vi "ToModelQueue_bac.vi"(7 "Enum":T1, 8 "error in (no error)":errorcluster) -> (0 "error out":errorcluster, 3 "queue out":refnum<queue>)   [LabVIEW 2021]
uses:
  QueueEnum.ctl
  ModelQueueCluster.ctl
  ToModelSourceEnum.ctl
  FromTCPCluster.ctl
  ToModelFromTCPMessage.ctl
  FormControllerToMOdelCluster.ctl
  ToModelFromControllerEnum.ctl
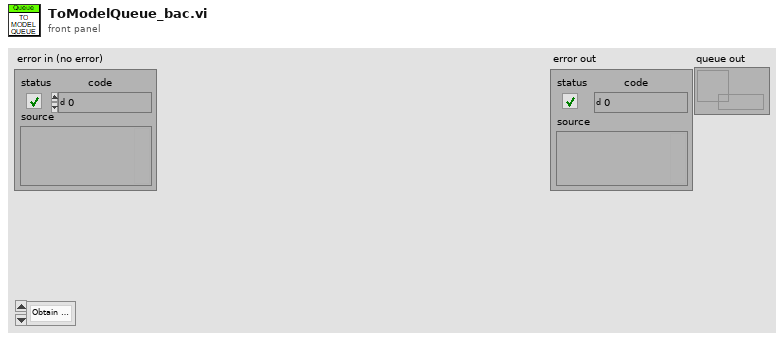
[diagram p1: front panel]
types:
  T1 = typedef "QueueEnum.ctl" = enum16{"Obtain Queue", "Get Queue Ref", "Flush Queue", "Release Queue"}
  T2 = typedef "ModelQueueCluster.ctl" = cluster{T3, "FromTCPCluster":T4, "FromControllerCluster":T6}
  T3 = typedef "ToModelSourceEnum.ctl" = enum16{"TCP", "Controller"}
  T4 = typedef "FromTCPCluster.ctl" = cluster{"Message":T5, "Data":string, "StatusOK?":bool}
  T5 = typedef "ToModelFromTCPMessage.ctl" = enum16{"Exit", "DataWritten", "DataReceived", "Timeout", "UnableToConnect", "Disconnected", "Connected"}
  T6 = typedef "FormControllerToMOdelCluster.ctl" = cluster{"Enum":T7, "IP Address":string, "Remote Port":u16}
  T7 = typedef "ToModelFromControllerEnum.ctl" = enum16{"Disconnect", "Connect"}
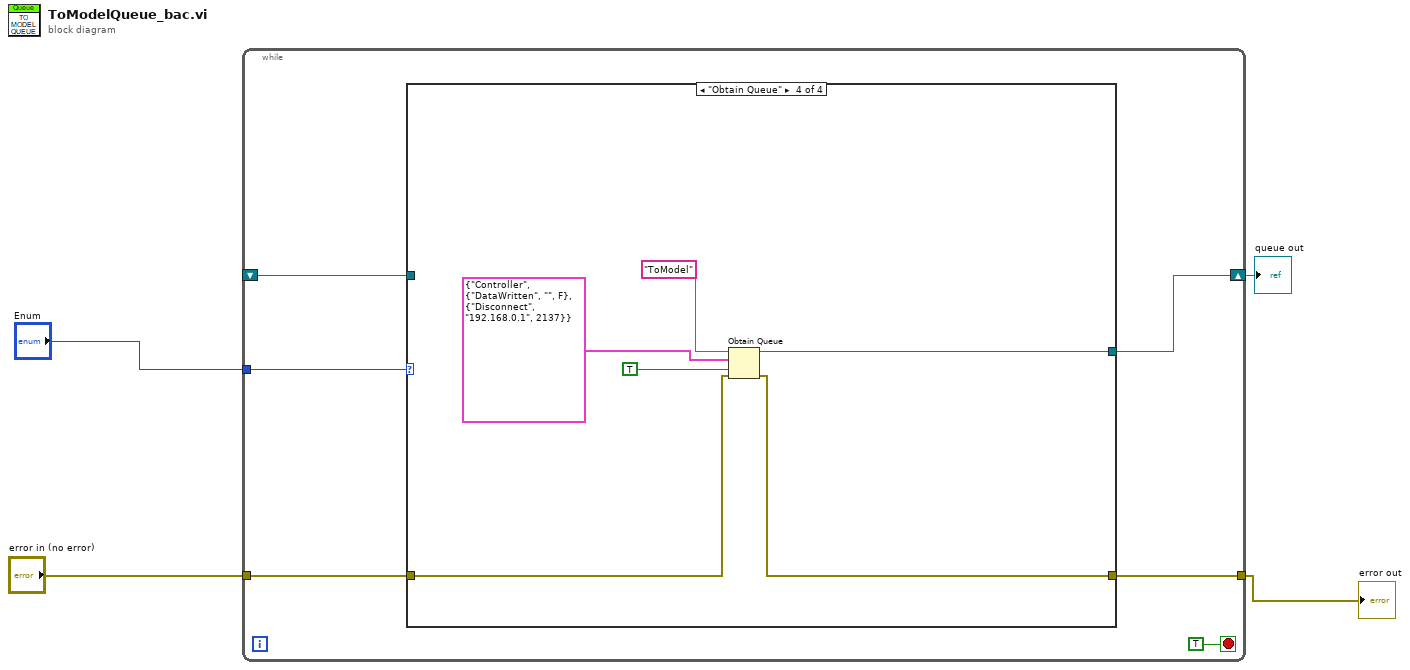
[diagram p0: block diagram]
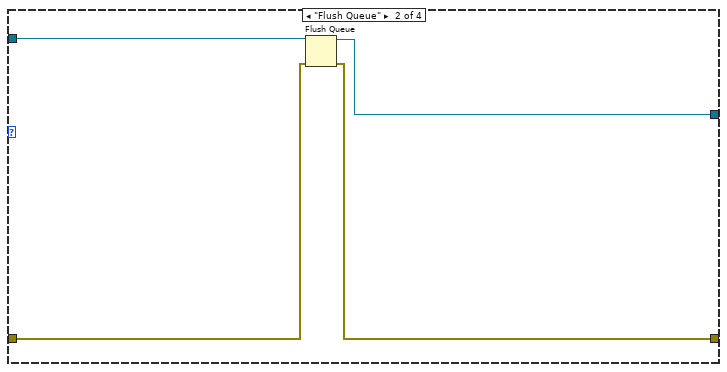
[diagram p3: hidden frame]
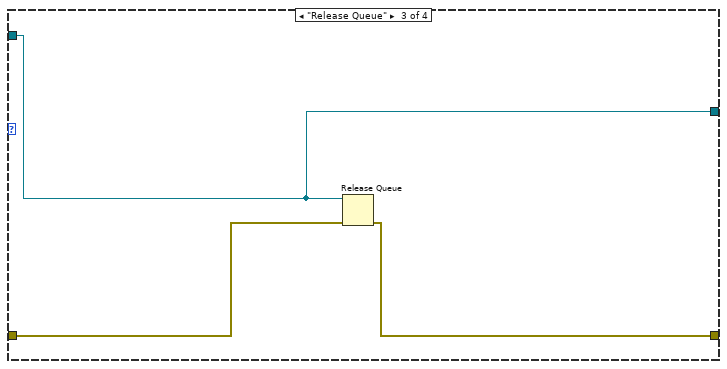
[diagram p4: hidden frame]
diagram:
  n1 = while {
    tunnel: "error in (no error)" -> [w8]
    tunnel: [w7] -> w3
    tunnel: "Enum" -> [w9]
    shift-right: [w6] -> w1
    shift-left: _ -> [w5]
    stop <- TRUE stop-if-true
    n2 = case shown="\"Obtain Queue\"" w9 {
      tunnel: w8 -> [w11 w15 w19 w24]
      tunnel: [w11 w14 w18 w22] -> w7
      tunnel: [w12 w13 w17 w21] -> w6
      tunnel: w5 -> [w12 w16 w17 _]
      frame "Get Queue Ref", Default {
      }
      frame "Flush Queue" {
        n3 = Flush Queue(queue=w16, error in (no error)=w15) -> (queue out=w13:refnum<queue>, error out=w14:errorcluster)  [unwired: 1 out]
      }
      frame "Release Queue" {
        n4 = Release Queue(queue=w17, error in (no error)=w19) -> (error out=w18:errorcluster)  [unwired: 1 in, 2 out]
      }
      frame "Obtain Queue" {
        n5 = Obtain Queue(name (unnamed)="ToModel", element data type=T2 {enum."Controller", "FromTCPCluster"={"Message"=enum."DataWritten", "Data"="", "StatusOK?"=FALSE}, "FromControllerCluster"={"Enum"=enum."Disconnect", "IP Address"="192.168.0.1", "Remote Port"=2137}}, create if not found? (T)=TRUE, error in (no error)=w24) -> (queue out=w21:refnum<queue>, error out=w22:errorcluster)  [unwired: 1 in, 1 out]
      }
    }
  }
  "error out" <- w3
  "queue out" <- w1
